vi "write_attributes.vi"(8 "error in (no error)":errorcluster, 10 "attributes":T1, 11 "ExtraTreesClassifier in":refnum<class "ExtraTreesClassifier.lvclass">) -> (0 "error out":errorcluster, 3 "ExtraTreesClassifier out":refnum<class "ExtraTreesClassifier.lvclass">)   [LabVIEW 2020, in "ExtraTreesClassifier.lvclass"]
uses:
  ExtraTreesClassifier.lvclass
  Controls/extra_trees_classifier_attributes.ctl
  ExtraTreesClassifier.lvclass/ExtraTreesClassifier.ctl
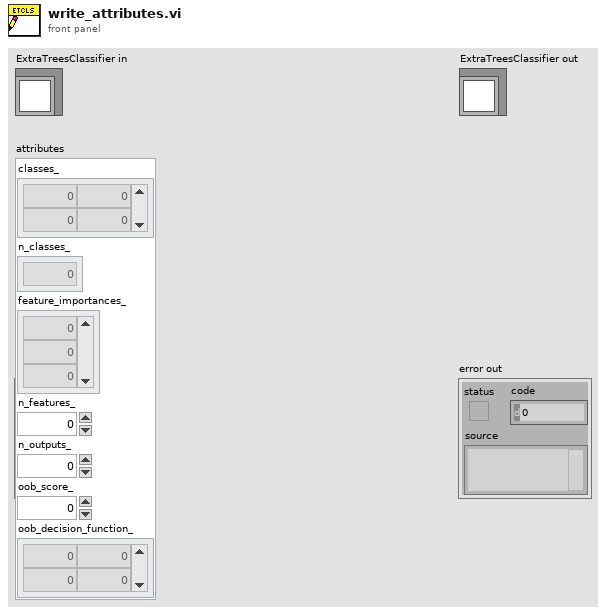
[diagram p1: front panel]
types:
  T1 = typedef "extra_trees_classifier_attributes.ctl" = cluster{"classes_":dbl[][], "n_classes_":dbl[], "feature_importances_":dbl[], "n_features_":dbl, "n_outputs_":dbl, "oob_score_":dbl, "oob_decision_function_":dbl[][]}
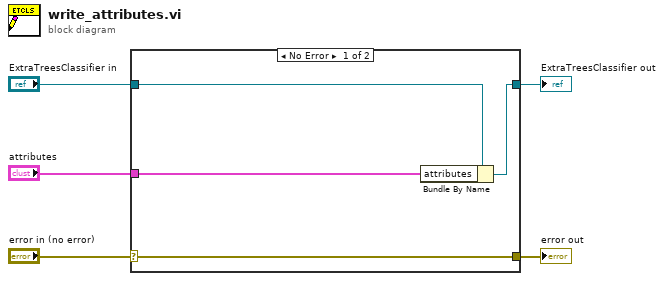
[diagram p0: block diagram]
diagram:
  n1 = case shown="No Error" "error in (no error)" {
    selector: "error in (no error)" -> [w9 w10]
    tunnel: [w9 w10] -> w4
    tunnel: [w7 w11] -> w2
    tunnel: "ExtraTreesClassifier in" -> [w8 w11]
    tunnel: "attributes" -> [w6 _]
    frame No Error {
      n2 = Bundle By Name(cluster=w8, "attributes"=w6) -> (w7:refnum<class "ExtraTreesClassifier.lvclass">)
    }
    frame Error {
    }
  }
  "error out" <- w4
  "ExtraTreesClassifier out" <- w2
